vi "Set Hardware Configuration File Path.vi"(8 "error in":errorcluster, 10 "Path":path, 11 "Configuration files Ref":T1 format="%.0x") -> (0 "error out":errorcluster, 3 "Configuration files Ref out":T1 format="%.0x")   [LabVIEW 2020, in "Ballard ARINC 429 Scripting.lvlib"]
uses:
  Ballard ARINC 429 Scripting.lvlib
  <vilib>/NI VeriStand/Custom Device API/Custom Device Item Ref.ctl
  <vilib>/NI VeriStand/Custom Device API/Dependent File Optional Info.ctl
  Constants.vi
  <vilib>/NI VeriStand/Custom Device API/Set Item Property (Dependent File).vi
  <vilib>/NI VeriStand/Custom Device API/Custom Device API.lvlib
  System Explorer/Implementation/Implementation.lvlib
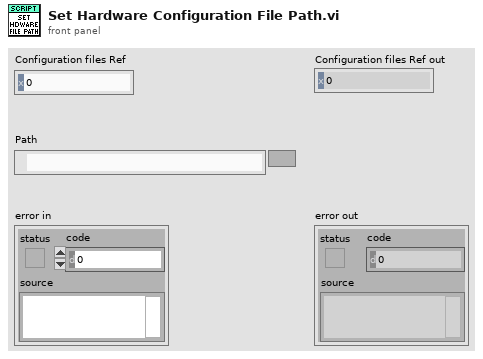
[diagram p1: front panel]
types:
  T1 = typedef "Custom Device API.lvlib/Custom Device Item Ref.ctl" = u64
  T2 = typedef "Custom Device API.lvlib/Dependent File Optional Info.ctl" = cluster{"Version":string, "RTDestination":path, "ForceDownload":bool, "SupportedTarget":string, "MD5":string}
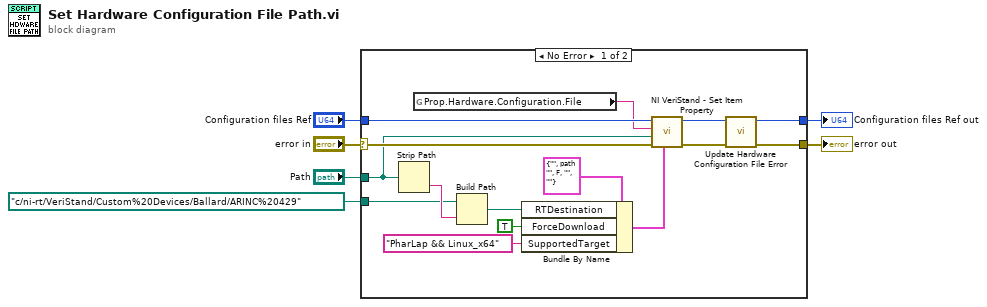
[diagram p0: block diagram]
diagram:
  n1 = case shown="No Error" "error in" {
    selector: "error in" -> [w20 w23]
    tunnel: "Configuration files Ref" -> [w21 w22]
    tunnel: [w15 w23] -> w5
    tunnel: [w17 w22] -> w3
    tunnel: "Path" -> [w12 _]
    tunnel: path "c:/ni-rt/VeriStand/Custom%20Devices/Ballard/ARINC%20429" ("RTDestination") -> [w10 _]
    frame No Error {
      n2 = Strip Path(path=w12) -> (name=w11:string)  [unwired: 1 out]
      n3 = global read "Constants.vi" "Prop.Hardware.Configuration.File"() -> (w19:string)
      n4 = Build Path(base path=w10, name or relative path=w11) -> (appended path=w9:path)
      n5 = Bundle By Name(cluster=T2 {"Version"="", "RTDestination"=path "", "ForceDownload"=FALSE, "SupportedTarget"="", "MD5"=""} ("OptionalInfo"), "RTDestination"=w9, "ForceDownload"=TRUE, "SupportedTarget"="PharLap && Linux_x64") -> (w13:T2)
      n6 = call-poly <vilib>:"NI VeriStand - Set Item Property.vi"("OptionalInfo"=w13, "error in (no error)"=w20, "Path"=w12, "Property Name"=w19, "Item Ref in"=w21) -> ("error out"=w16:errorcluster, "Item Ref out"=w18:T1)  [unwired: 4 in, 1 out]
      n7 = call "Update Hardware Configuration File Error.vi"("error in"=w16, "Configuration files Ref"=w18) -> ("error out"=w15:errorcluster, "Configuration files Ref out"=w17:T1)  [unwired: 8 in]
    }
    frame Error {
    }
  }
  "error out" <- w5
  "Configuration files Ref out" <- w3
